vi "WebVGA server.vi"(9 "timeout ms (wait forever: -1)":i32=-1, 10 "port (25681)":u16=25681, 11 "Title (WebVGA interface)":string="WebVGA interface") -> (2 "remote port":u16, 3 "remote address":string)   [LabVIEW 2014]
uses:
  Global vars.vi
panel:
  out "my address":string
  out "error out":errorcluster
  out "HTTP request":string
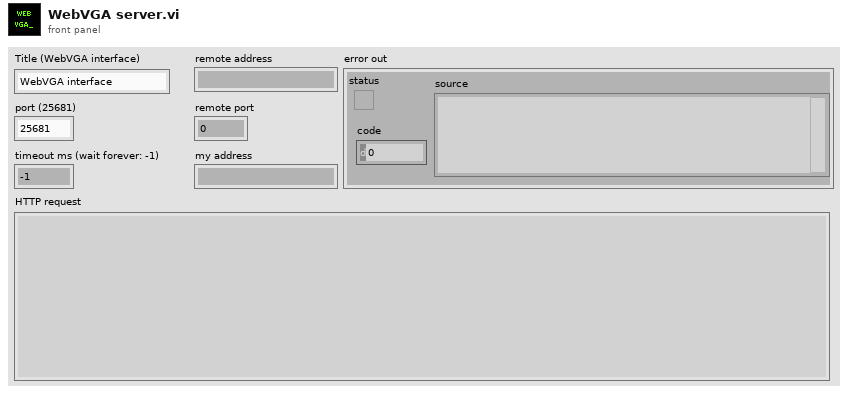
[diagram p1: front panel]
types:
  T1 = enum16{"Standard", "Buffered", "CRLF", "Immediate"}
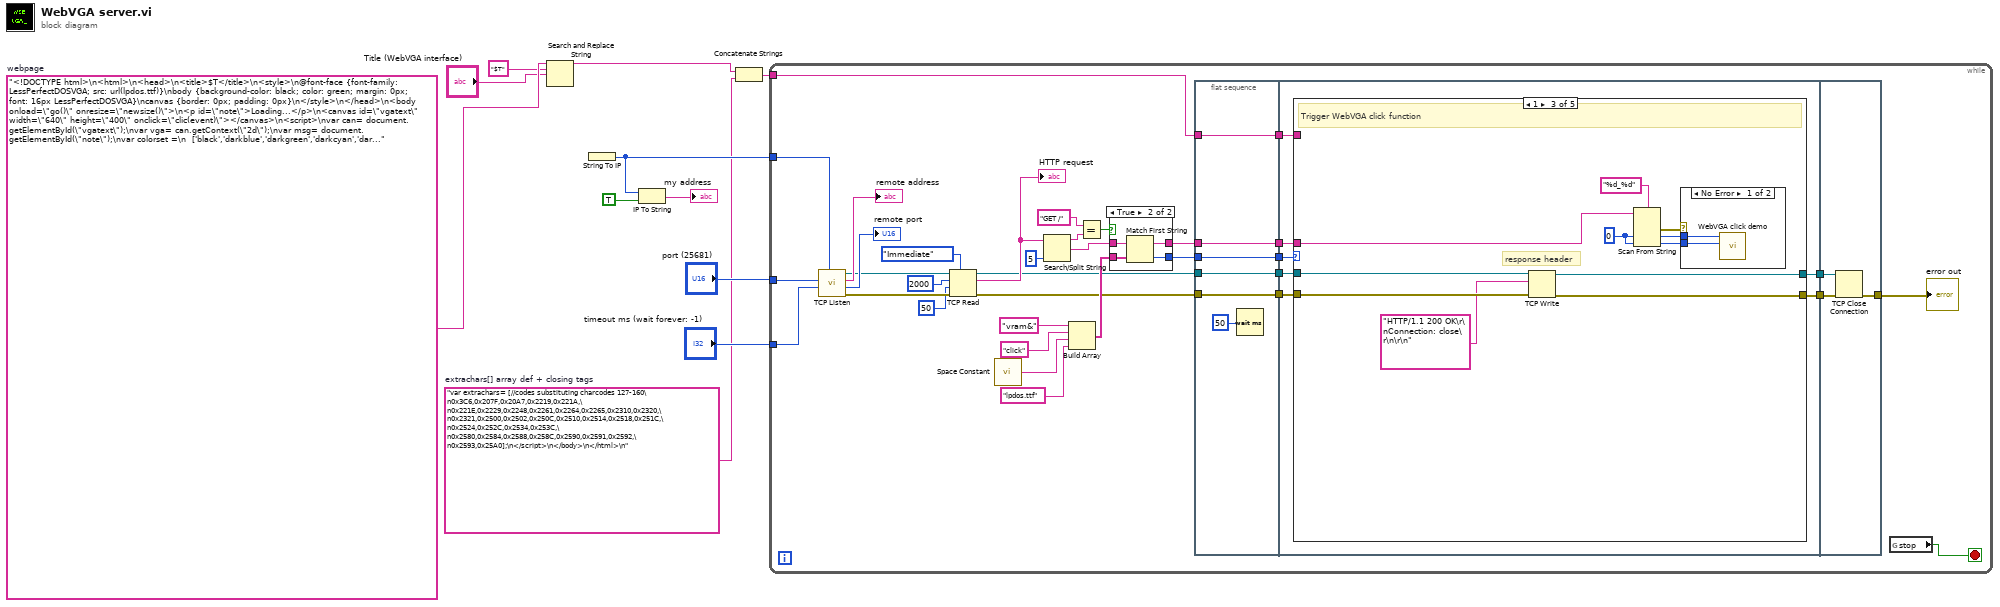
[diagram p0: block diagram]
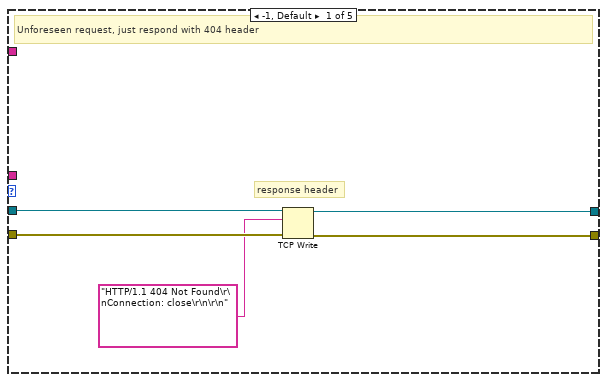
[diagram p2: hidden frame]
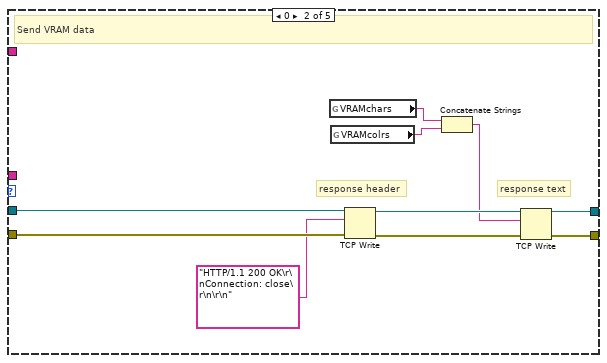
[diagram p3: hidden frame]
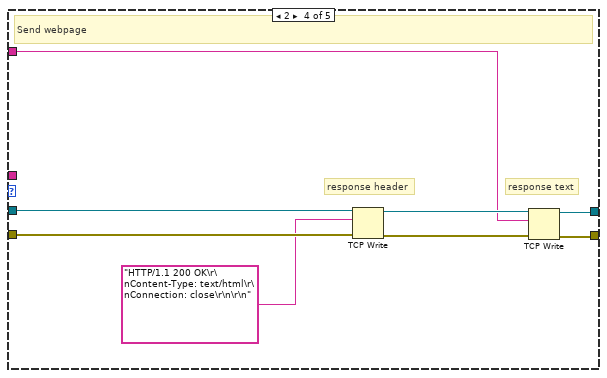
[diagram p5: hidden frame]
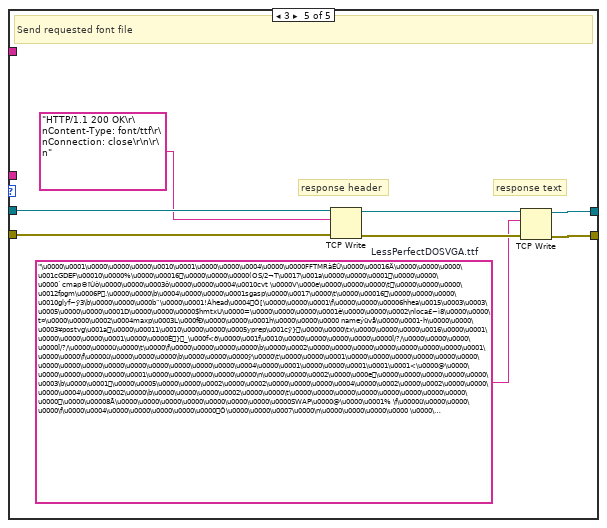
[diagram p6: hidden frame]
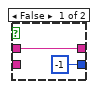
[diagram p7: hidden frame]
diagram:
  w1 = "var extrachars= [//codes substituting charcodes 127-160\n0x3C6,0x207F,0x20A7,0x2219,0x221A,\n0x221E,0x2229,0x2248,0x2261,0x2264,0x2265,0x2310,0x2320,\n0x2321,0x2500,0x2502,0x250C,0x2510,0x2514,0x2518,0x251C,\n0x2524,0x252C,0x2534,0x253C,\n0x2580,0x2584,0x2588,0x258C,0x2590,0x2591,0x2592,\n0x2593,0x25A0];\n</script>\n</body>\n</html>\n"  # extrachars[] array def + closing tags
  w9 = "<!DOCTYPE html>\n<html>\n<head>\n<title>$T</title>\n<style>\n@font-face {font-family: LessPerfectDOSVGA; src: url(lpdos.ttf)}\nbody {background-color: black; color: green; margin: 0px; font: 16px LessPerfectDOSVGA}\ncanvas {border: 0px; padding: 0px}\n</style>\n</head>\n<body onload=\"go()\" onresize=\"newsize()\">\n<p id=\"note\">Loading...</p>\n<canvas id=\"vgatext\" width=\"640\" height=\"400\" onclick=\"clic(event)\"></canvas>\n<script>\nvar can= document.getElementById(\"vgatext\");\nvar vga= can.getContext(\"2d\");\nvar msg= document.getElementById(\"note\");\nvar colorset =\n  ['black','darkblue','darkgreen','darkcyan','darkred','darkmagenta','saddlebrown','grey',\n   'dimgrey', 'blue', 'green', 'cyan', 'orangered', 'hotpink', 'yellow', 'white'];\nvar vram=\"\", charsize=16, charw=8, clock=0, colnum=[0,0];\n\nfunction go() { //at the beginning, execute go() every 3 sec until VRAM first loads\nvramupdate();\nif (vram==\"\") setTimeout(go, 3000)\nelse {\n  msg.style.display= \"none\"; //hide top <p>\n  newsize();\n  setInterval(vramupdate, 3300); //then update VRAM every 3.3 sec\n  setInterval(screfresh, 1000); //and refresh screen every sec\n}\n}\n\nfunction newsize() { //resizes canvas to fit window\nvar w = window.innerWidth\n  || document.documentElement.clientWidth\n  || document.body.clientWidth;\nvar h = window.innerHeight\n  || document.documentElement.clientHeight\n  || document.body.clientHeight;\nif (w/h > 1.6) charw= Math.max(8, Math.floor(h/50)) //limiting factor is window height\n  else charw= Math.max(8, Math.floor(w/80)); //limiting factor is window width\ncharsize= 2*charw;\ncan.width= 80*charw;\ncan.height= 25*charsize;\nvga.font= charsize+\"px LessPerfectDOSVGA\";\nvga.textBaseline= \"top\";\n}\n\nfunction vramupdate() { http_get(\"vram&nocache=\"+Math.random()*1e6) }\n\nfunction clic(event) {\nvar rect = can.getBoundingClientRect();\nvar xclic = event.clientX - rect.left;\nvar yclic = event.clientY - rect.top;\nvar row= Math.ceil((yclic+1)/charsize);\nvar col= Math.ceil((xclic+1)/charw);\nhttp_get(\"click\"+row+\"_\"+col+\"&nocache=\"+Math.random()*1e6);\n}\n\nfunction screfresh() {\nvar i, j, x, y, charcode, colbyte, ind=0;\nclock= 1-clock; //switches every sec between 0 and 1\nfor (i=0; i<25; i++) for (j=0; j<80; j++) { //cycle thru and print all 80x25 chars\n  x= j*charw;\n  y= i*charsize;\n  charcode= vram[ind];\n  if (charcode<32) charcode+= 0x254D //add some extra chars...\n  else if ((charcode>=127)&&(charcode<=160)) charcode= extrachars[charcode-127];\n  colbyte= vram[ind+2000];\n  colnum[1]= colbyte >> 4; //background color num\n  colnum[0]= colbyte & 15; //foreground color num\n  if (colnum[0]==colnum[1])\n    if (colnum[0] > 7) colnum[clock] -= 8  //flashing char (both bg&fg)\n    else if (clock==1) colnum[0] += 8 ; //blinking foreground only\n  vga.fillStyle= colorset[colnum[1]];\n  vga.fillRect(x,y,charw,charsize);\n  vga.fillStyle= colorset[colnum[0]];\n  vga.fillText(String.fromCharCode(charcode), x, y);\n  ind++;\n}\n}\n\nfunction http_get(that) { //sends HTTP GET request for that\nvar oReq = new XMLHttpRequest();\noReq.open(\"GET\", that, true);\noReq.responseType = \"arraybuffer\";\n//________\noReq.onload = function (oEvent) {\nvar buf = oReq.response; // Note: not oReq.responseText\nif (buf.byteLength==4000) vram = new Uint8Array(buf);\n}; //________\noReq.send(null);\n}\n// add var defs + closing tags\n"  # webpage
  n1 = Search and Replace String(input string=w9, search string="$T" ("string"), replace string="Title (WebVGA interface)") -> (result string=w6:string)  [unwired: 5 in, 3 out]
  n2 = String To IP() -> (0:w4:u32)  [unwired: 1 in]
  n3 = IP To String(1:TRUE ("dot notation? (F)"), 2:w4) -> (0:→"my address":string)
  n4 = Concatenate Strings(w6, w1) -> (w2:string)
  n5 = while {
    tunnel: "port (25681)" -> [w45]
    tunnel: "timeout ms (wait forever: -1)" -> [w42]
    tunnel: w2 -> [w27]
    tunnel: w4 -> [w26]
    stop <- w46 stop-if-true
    n6 = call <vilib>:"TCP Listen.vi"("net address"=w26, "timeout ms (wait forever: -1)"=w42, "port"=w45) -> ("error out"=w40:errorcluster, "remote port"=→"remote port":u16, "remote address"=→"remote address":string, "connection ID"=w41:refnum<k5>)  [unwired: 4 in, 1 out]
    n7 = TCP Read(connection ID=w41, bytes to read=2000, error in (no error)=w40, 7:T1."Immediate" ("mode (standard)"), 9:50 ("bytes to read")) -> (connection ID out=w14:refnum<k5>, data out=w23:string, error out=w22:errorcluster)
    "HTTP request" <- w23
    n8 = call <vilib>:"Space Constant.vi"() -> ("String"=w36:string)
    n9 = Search/Split String(string=w23, offset (0)=5) -> (substring before match=w32:string, match + rest of string=w29:string)  [unwired: 1 in, 1 out]
    n10 = Build Array("vram&", "click", w36, "lpdos.ttf") -> (w28:string[])
    n11 = Equal?(x="GET /", y=w32) -> (x = y?=w30:bool)
    n12 = case shown="True" w30 {
      tunnel: [-1 ("index") w112] -> w39
      tunnel: [w108 w111] -> w34
      tunnel: w29 -> [w108 w110]
      tunnel: w28 -> [_ w109]
      frame False {
      }
      frame True {
        n13 = Match First String(2:w109, 3:w110) -> (0:w112:i32, 1:w111:string)
      }
    }
    n14 = flat-sequence {
      tunnel: w27 -> [w48]
      tunnel: w34 -> [w49]
      tunnel: w22 -> [w50]
      tunnel: w14 -> [w51]
      tunnel: w39 -> [w52]
      tunnel: [w52] -> w19
      tunnel: [w51] -> w18
      tunnel: [w50] -> w17
      tunnel: [w49] -> w16
      tunnel: [w48] -> w15
      tunnel: [w54] -> w21
      tunnel: [w53] -> w20
      tunnel: w19 -> [w59]
      tunnel: w18 -> [w58]
      tunnel: w17 -> [w57]
      tunnel: w16 -> [w56]
      tunnel: w15 -> [w55]
      tunnel: [w105] -> w25
      tunnel: w21 -> [w104]
      tunnel: w20 -> [w106]
      frame #0 {
        n15 = Wait (ms)(milliseconds to wait=u32 50) -> ()  [unwired: 1 out]
      }
      frame #1 {
        n16 = case shown="1" w59 {
          tunnel: w58 -> [w64 w74 w85 w95 w103]
          tunnel: w57 -> [w63 w73 w84 w94 w102]
          tunnel: w56 -> [_ _ w80 _ _]
          tunnel: w55 -> [_ _ _ w89 _]
          tunnel: [w62 w70 w83 w91 w99] -> w54
          tunnel: [w61 w69 w82 w90 w98] -> w53
          frame -1, Default {
            # "response header"
            # "Unforeseen request, just respond with 404 header"
            n17 = TCP Write(connection ID=w64, data in="HTTP/1.1 404 Not Found\r\nConnection: close\r\n\r\n", error in (no error)=w63) -> (connection ID out=w62:refnum<k5>, error out=w61:errorcluster)  [unwired: 1 in, 1 out]
          }
          frame 0 {
            # "response text"
            # "response header"
            # "Send VRAM data"
            n18 = global read "Global vars.vi" "VRAMchars"() -> (w67:string)
            n19 = global read "Global vars.vi" "VRAMcolrs"() -> (w68:string)
            n20 = TCP Write(connection ID=w74, data in="HTTP/1.1 200 OK\r\nConnection: close\r\n\r\n", error in (no error)=w73) -> (connection ID out=w72:refnum<k5>, error out=w71:errorcluster)  [unwired: 1 in, 1 out]
            n21 = Concatenate Strings(w67, w68) -> (w66:string)
            n22 = TCP Write(connection ID=w72, data in=w66, error in (no error)=w71) -> (connection ID out=w70:refnum<k5>, error out=w69:errorcluster)  [unwired: 1 in, 1 out]
          }
          frame 1 {
            w75 = u8 0 ("default value 1")
            # "response header"
            # "Trigger WebVGA click function"
            n23 = TCP Write(connection ID=w85, data in="HTTP/1.1 200 OK\r\nConnection: close\r\n\r\n", error in (no error)=w84) -> (connection ID out=w83:refnum<k5>, error out=w82:errorcluster)  [unwired: 1 in, 1 out]
            n24 = Scan From String(format string="%d_%d", input string=w80, default 1=w75, default 2=w75) -> (error out=w78:errorcluster, output 1=w77:u8, output 2=w76:u8)  [unwired: 2 in, 2 out]
            n25 = case shown="No Error" w78 {
              tunnel: w77 -> [w87 _]
              tunnel: w76 -> [w86 _]
              frame No Error {
                n26 = call "WebVGA click demo.vi"("Column"=w86, "Row"=w87) -> ()  [unwired: 10 in]
              }
              frame Error {
              }
            }
          }
          frame 2 {
            # "response text"
            # "response header"
            # "Send webpage"
            n27 = TCP Write(connection ID=w95, data in="HTTP/1.1 200 OK\r\nContent-Type: text/html\r\nConnection: close\r\n\r\n", error in (no error)=w94) -> (connection ID out=w93:refnum<k5>, error out=w92:errorcluster)  [unwired: 1 in, 1 out]
            n28 = TCP Write(connection ID=w93, data in=w89, error in (no error)=w92) -> (connection ID out=w91:refnum<k5>, error out=w90:errorcluster)  [unwired: 1 in, 1 out]
          }
          frame 3 {
            w97 = "\u0000\u0001\u0000\u0000\u0000\u0010\u0001\u0000\u0000\u0004\u0000\u0000FFTMRàÉÛ\u0000\u00016Ä\u0000\u0000\u0000\u001cGDEF\u00010\u0000%\u0000\u00016\u0000\u0000\u0000(OS/2¬T\u0017\u001a\u0000\u0000\u0001\u0000\u0000\u0000`cmap©ïÙò\u0000\u0000\u0003ô\u0000\u0000\u0004\u0010cvt \u0000V\u000e\u0000\u0000\u0000\t\u0000\u0000\u0000\u0012fpgm\u0006P.\u0000\u0000\b\u0004\u0000\u0000\u0001sgasp\u0000\u0017\u0000\t\u0000\u00016\u0000\u0000\u0000\u0010glyf~ÿ3\b\u0000\u0000\u000b¨\u0000\u0001!Àhead\u0004Ó[\u0000\u0000\u0001\f\u0000\u0000\u00006hhea\u0015\u0003\u0003\u0005\u0000\u0000\u0001D\u0000\u0000\u0000$hmtxU\u0000=\u0000\u0000\u0000\u0001è\u0000\u0000\u0002\nloca£~ì8\u0000\u0000\t¤\u0000\u0000\u0002\u0004maxp\u0003L\u000fÐ\u0000\u0000\u0001h\u0000\u0000\u0000 nameýüvå\u0000\u0001-h\u0000\u0000\u0003¥postvg\u001a\u0000\u00011\u0010\u0000\u0000\u0005yprep\u001cÿ}\u0000\u0000\tx\u0000\u0000\u0000\u0016\u0000\u0001\u0000\u0000\u0000\u0001\u0000\u0000È}_\u000f<õ\u0000\u001f\u0010\u0000\u0000\u0000\u0000\u0000Î/?/\u0000\u0000\u0000\u0000Î/?/\u0000\u0000ü\u0000\t\u0000\f\u0000\u0000\u0000\u0000\b\u0000\u0002\u0000\u0000\u0000\u0000\u0000\u0000\u0000\u0001\u0000\u0000\f\u0000ü\u0000\u0000\u0000\b\u0000\u0000\u0000ÿ\u0000\t\u0000\u0000\u0001\u0000\u0000\u0000\u0000\u0000\u0000\u0000\u0000\u0000\u0000\u0000\u0000\u0000\u0000\u0000\u0004\u0000\u0001\u0000\u0000\u0001\u0001\u0001<\u0000@\u0000\u0000\u0000\u0000\u0000\u0001\u0000\u0000\u0000\u0000\u0000\n\u0000\u0000\u0002\u0000\u000e\u0000\u0000\u0000\u0000\u0000\u0003\b\u0000\u0001\u0000\u0005\u0000\u0000\u0002\u0000\u0002\u0000\u0000\u0000\u0004\u0000\u0002\u0000\u0002\u0000\u0000\u0000\u0004\u0000\u0002\u0000\b\u0000\u0000\u0000\u0002\u0000\u0000\t\u0000\u0000\u0000\u0000\u0000\u0000\u0000\u0000\u0000\u0000\u00008Ã\u0000\u0000\u0000\u0000\u0000\u0000\u0000\u0000SWAP\u0000@\u0000\u0001% \f\u0000ü\u0000\u0000\u0000\f\u0000\u0004\u0000\u0000\u0000\u0000\u0000Ô\u0000\u0000\u0007\u0000\n\u0000\u0000\u0000\u0000 \u0000\u0001\b\u0000\u0000\u0000\u0000\u0000\u0000\u0000\b\u0000\u0000\u0000\b\u0000\u0000\u0000\u0000\u0000\u0000\u0000\u0000\u0000\u0000\u0000\u0000\u0000\u0002\u0000\u0000\u0000\u0001\u0000\u0000\u0000\u0000\u0000\u0000\u0000\u0000\u0000\u0000\u0000\u0000\u0000\u0000\u0000\u0001\u0000\u0001\u0000\u0000\u0000\u0000\u0000\u0000\u0000\u0001\u0000\u0001\u0000\u0001\u0000\u0000\u0000\u0000\u0000\u0000\u0000\u0000\u0000\u0000\u0000\u0000\u0000\u0000\u0000\u0002\u0000\u0001\u0000\u0000\u0000\u0000\u0000\u0000\u0000\u0000\u0000\u0001\u0000\u0002\u0000\u0002\u0000\u0000\u0000\u0001\u0000\u0002\u0000\u0000\u0000\u0003\u0000\u0000\u0000\u0000\u0000\u0001\u0000\u0000\u0000..."  # LessPerfectDOSVGA.ttf
            # "response text"
            # "response header"
            # "Send requested font file"
            n29 = TCP Write(connection ID=w103, data in="HTTP/1.1 200 OK\r\nContent-Type: font/ttf\r\nConnection: close\r\n\r\n", error in (no error)=w102) -> (connection ID out=w101:refnum<k5>, error out=w100:errorcluster)  [unwired: 1 in, 1 out]
            n30 = TCP Write(connection ID=w101, data in=w97, error in (no error)=w100) -> (connection ID out=w99:refnum<k5>, error out=w98:errorcluster)  [unwired: 1 in, 1 out]
          }
        }
      }
      frame #2 {
        n31 = TCP Close Connection(connection ID=w104, error in (no error)=w106) -> (error out=w105:errorcluster)  [unwired: 1 in, 1 out]
      }
    }
    n32 = global read "Global vars.vi" "stop"() -> (w46:bool)
    "error out" <- w25
  }
